vi "Add Line.vi"(8 "error in (no error)":errorcluster, 10 "Line":refnum<class "Line.lvclass">, 11 "Method in":refnum<class "Method.lvclass">) -> (0 "error out":errorcluster, 3 "Method out":refnum<class "Method.lvclass">)   [LabVIEW 2017, in "Cobertura.lvlib" / "Method.lvclass"]
uses:
  Method.lvclass
  Line/Line.lvclass
  Method.lvclass/Method.ctl
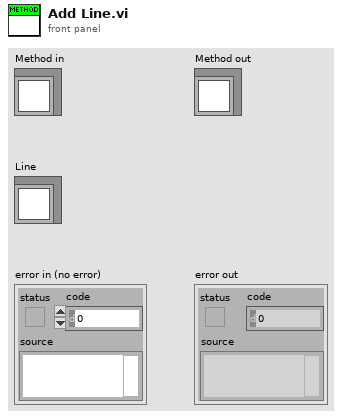
[diagram p1: front panel]
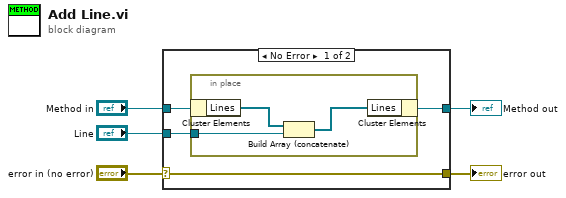
[diagram p0: block diagram]
diagram:
  n1 = case shown="No Error" "error in (no error)" {
    selector: "error in (no error)" -> [w9 w14]
    tunnel: [w9 w14] -> w4
    tunnel: [w7 w13] -> w2
    tunnel: "Method in" -> [w8 w13]
    tunnel: "Line" -> [w6 _]
    frame No Error {
      n2 = in-place {
        in-place-border: w6 -> [w10]
        n3 = in-place-cluster #1(w8) -> ("Lines"=w12:refnum<class "Line.lvclass">[])
        n4 = Build Array (concatenate)(w12, w10) -> (w11:refnum<class "Line.lvclass">[])
        n5 = in-place-cluster #1("Lines"=w11) -> (w7:refnum<class "Method.lvclass">)
      }
    }
    frame Error {
    }
  }
  "error out" <- w4
  "Method out" <- w2
